vi "SRV_PM_App Initializaton Routine.vi"(6 "Packet Mode Enable (T)":bool=TRUE, 7 "Read Response (F)":bool, 8 "error in (no error)":errorcluster, 11 "connection ID":refnum<k5>) -> (0 "error out":errorcluster, 1 "Command Sent":string, 3 "connection ID out":refnum<k5>, 5 "Response":string)   [LabVIEW 2009]
uses:
  TCP_Communication/SRV_TCP Settings.ctl
  TCP_Communication/SRV_Package Methods.ctl
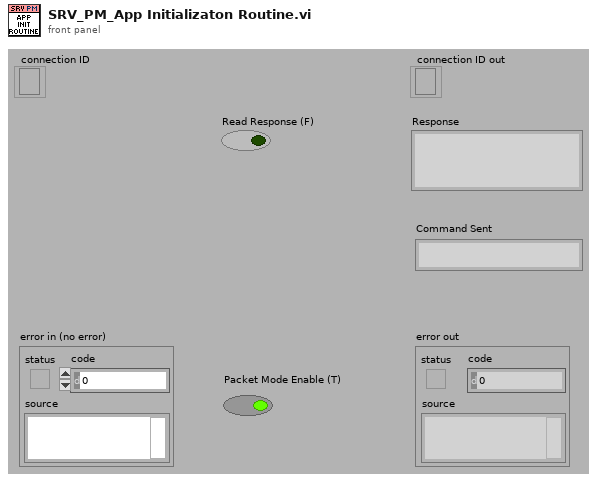
[diagram p1: front panel]
types:
  T1 = typedef "SRV_TCP Settings.ctl" = cluster{"Method":T2, "bytes to read":i32, "timeout ms (1000)":i32}
  T2 = typedef "SRV_Package Methods.ctl" = enum16{"General", "Standard", "CRLF", "Image", "HTML"}
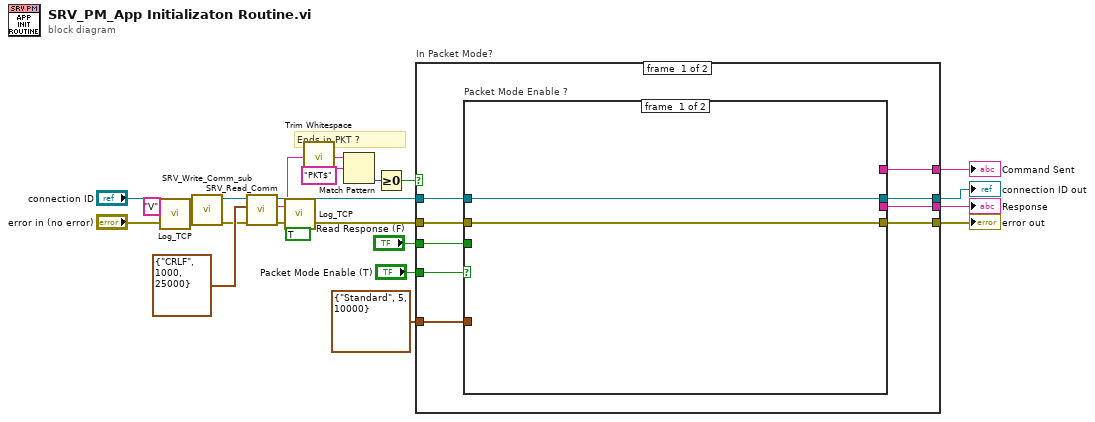
[diagram p0: block diagram]
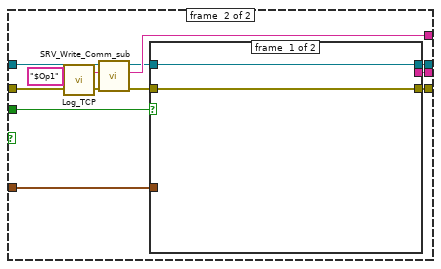
[diagram p2: hidden frame]
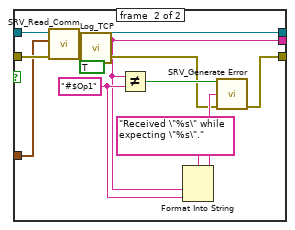
[diagram p3: hidden frame]
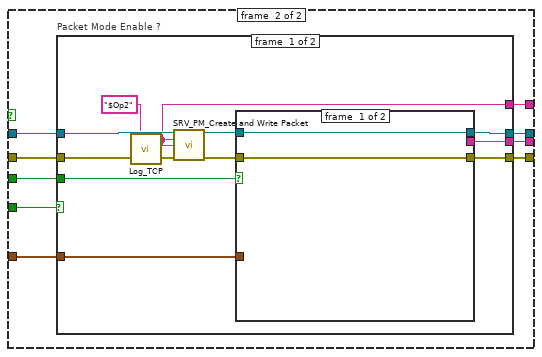
[diagram p4: hidden frame]
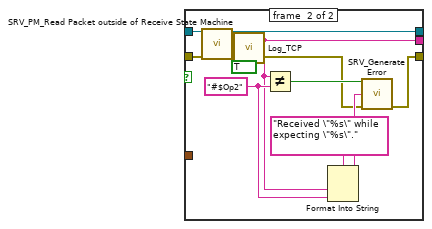
[diagram p5: hidden frame]
diagram:
  # "Ends in PKT ?"
  n1 = call "Log_TCP.vi"("Data"="V" ("Command Sent"), "error in (no error)"="error in (no error)") -> ("Data dup"=w5:string, "error out"=w7:errorcluster)  [unwired: 12 in]
  n2 = call "SRV_Write_Comm_sub.vi"("error in (no error)"=w7, "Command Sent"=w5, "SRV In"="connection ID") -> ("error out"=w9:errorcluster, "SRV Out"=w22:refnum<k5>)  [unwired: 6 in, 1 out]
  n3 = call "SRV_Read_Comm.vi"("error in (no error)"=w9, "TCP Settings"=T1 {"Method"=enum."CRLF", "bytes to read"=1000, "timeout ms (1000)"=25000}, "SRV In"=w22) -> ("error out"=w4:errorcluster, "Data out"=w2:string, "SRV Out"=w16:refnum<k5>)  [unwired: 6 in]
  n4 = call "Log_TCP.vi"("Data"=w2, "error in (no error)"=w4, "Response? (F: LV Writes)"=TRUE) -> ("error out"=w3:errorcluster)  [unwired: 11 in, 1 out]
  n5 = call <vilib>:"Trim Whitespace.vi"("string"=w2) -> ("trimmed string"=w21:string)  [unwired: 1 in]
  n6 = Match Pattern(string=w21, regular expression="PKT$") -> (offset past match=w19:i32)  [unwired: 1 in, 3 out]
  n7 = Greater Or Equal To 0?(x=w19) -> (x >= 0?=w18:bool)
  n8 = case "In Packet Mode?" shown="False" w18 {
    tunnel: w3 -> [w33 w72]
    tunnel: "Packet Mode Enable (T)" -> [w29 w73]
    tunnel: [w32 w71] -> w15
    tunnel: w16 -> [w30 w70]
    tunnel: [w31 w69] -> w14
    tunnel: [w28 w68] -> w13
    tunnel: "Read Response (F)" -> [w25 w67]
    tunnel: [w27 w66] -> w11
    tunnel: T1 {"Method"=enum."Standard", "bytes to read"=5, "timeout ms (1000)"=10000} ("TCP Settings") -> [w26 w65]
    frame #0 {
      n9 = case "Packet Mode Enable ?" shown="True" w29 {
        tunnel: w33 -> [w34 w39]
        tunnel: [w34 w44] -> w32
        tunnel: w30 -> [w35 w48]
        tunnel: [w35 w45] -> w31
        tunnel: [_ w47] -> w28
        tunnel: [_ w46] -> w27
        tunnel: w26 -> [_ w41]
        tunnel: w25 -> [_ w40]
        frame #0 {
        }
        frame #1 {
          n10 = call "Log_TCP.vi"("Data"="$Op1", "error in (no error)"=w39) -> ("Data dup"=w36:string, "error out"=w38:errorcluster)  [unwired: 12 in]
          n11 = call "SRV_Write_Comm_sub.vi"("error in (no error)"=w38, "Command Sent"=w36, "SRV In"=w48) -> ("error out"=w43:errorcluster, "Command Sent dup"=w47:string, "SRV Out"=w42:refnum<k5>)  [unwired: 6 in]
          n12 = case shown="True" w40 {
            tunnel: w43 -> [w49 w64]
            tunnel: [w49 w56] -> w44
            tunnel: w42 -> [w50 w63]
            tunnel: [w50 w62] -> w45
            tunnel: w41 -> [_ w61]
            tunnel: [_ w52] -> w46
            frame #0 {
            }
            frame #1 {
              w58 = "#$Op1" ("y")
              n13 = call "SRV_Read_Comm.vi"("error in (no error)"=w64, "TCP Settings"=w61, "SRV In"=w63) -> ("error out"=w55:errorcluster, "Data out"=w53:string, "SRV Out"=w62:refnum<k5>)  [unwired: 6 in]
              n14 = call "Log_TCP.vi"("Data"=w53, "error in (no error)"=w55, "Response? (F: LV Writes)"=TRUE) -> ("Data dup"=w52:string, "error out"=w54:errorcluster)  [unwired: 11 in]
              n15 = Not Equal?(x=w52, y=w58) -> (x != y?=w60:bool)
              n16 = Format Into String(format string="Received \"%s\" while expecting \"%s\".", w52, w58) -> (resulting string=w57:string)  [unwired: 2 in, 1 out]
              n17 = call "SRV_Generate Error.vi"("status (T)"=w60, "Message"=w57, "error in (no error)"=w54) -> ("error out"=w56:errorcluster)  [unwired: 12 in]
            }
          }
        }
      }
    }
    frame #1 {
      n18 = case "Packet Mode Enable ?" shown="False" w73 {
        tunnel: w72 -> [w76 w102]
        tunnel: [w83 w102] -> w71
        tunnel: w70 -> [w85 w101]
        tunnel: [w81 w101] -> w69
        tunnel: [w74 _] -> w68
        tunnel: w67 -> [w80 _]
        tunnel: [w79 _] -> w66
        tunnel: w65 -> [w78 _]
        frame #0 {
          n19 = call "Log_TCP.vi"("Data"="$Op2", "error in (no error)"=w76) -> ("Data dup"=w74:string, "error out"=w77:errorcluster)  [unwired: 12 in]
          n20 = call "SRV_PM_Create and Write Packet.vi"("SRV ref"=w85, "Command Type"=w74, "Data String"=w74, "error in (no error)"=w77) -> ("SRV ref out"=w82:refnum<k5>, "error out"=w84:errorcluster)  [unwired: 10 in]
          n21 = case shown="True" w80 {
            tunnel: w84 -> [w86 w95]
            tunnel: [w86 w100] -> w83
            tunnel: w82 -> [w87 w94]
            tunnel: [w87 w93] -> w81
            tunnel: w78 -> [_ _]
            tunnel: [_ w89] -> w79
            frame #0 {
            }
            frame #1 {
              w97 = "#$Op2" ("y")
              n22 = call "SRV_PM_Read Packet outside of Receive State Machine.vi"("SRV"=w94, "error in (no error)"=w95) -> ("SRV out"=w93:refnum<k5>, "Packet Data Field String"=w90:string, "error out"=w92:errorcluster)  [unwired: 9 in, 2 out]
              n23 = call "Log_TCP.vi"("Data"=w90, "error in (no error)"=w92, "Response? (F: LV Writes)"=TRUE) -> ("Data dup"=w89:string, "error out"=w91:errorcluster)  [unwired: 11 in]
              n24 = Not Equal?(x=w89, y=w97) -> (x != y?=w99:bool)
              n25 = Format Into String(format string="Received \"%s\" while expecting \"%s\".", w89, w97) -> (resulting string=w96:string)  [unwired: 2 in, 1 out]
              n26 = call "SRV_Generate Error.vi"("status (T)"=w99, "Message"=w96, "error in (no error)"=w91) -> ("error out"=w100:errorcluster)  [unwired: 12 in]
            }
          }
        }
        frame #1 {
        }
      }
    }
  }
  "connection ID out" <- w14
  "error out" <- w15
  "Command Sent" <- w13
  "Response" <- w11
